vi "Measurement UI.vi"() -> ()   [LabVIEW 2021, in "Quiescent Current_Channel Ganging_UI.lvlib"]
uses:
  Quiescent Current_Channel Ganging_UI.lvlib
panel:
  in  "MeasGraphs":enum32{"Q Current", "Hidden Controls"}(tab)
  out "QCurrentGraph(V/A)":T1(graph)
  in  "Source voltage pole-zero ratio":dbl=2.0
  in  "Source voltage compensation frequency":dbl=3530.0
  in  "Source voltage gain bandwidth":dbl=2000.0
  out "Q current minimum":dbl
  out "Q current maximum":dbl
  out "Ganged q currents":dbl[](array[numeric]) caption="Q currents"
  out "Ganged source voltages":dbl[](array[numeric]) caption="Source voltages"
  in  "Source slave resource names":string[](array[string])
  in  "Source master resource name":string
  out "MeasTable":string[][](table)
  in  "MeasConfigurations":enum32{"Measurement Config", "Source Config"}(tab)=enum."Source Config"
  in  "Source delay":dbl=0.005 caption="SOURCE DELAY" format="%.3ps"
  in  "DUT setup time":dbl=1.0 caption="DUT SETUP TIME" format="%.3ps"
  in  "Aperture time":dbl=0.005 caption="APERTURE TIME" format="%.3ps"
  in  "PPSSlaveResourceNames":refnum<k15>[](array[refnum]) caption="SLAVE RESOURCE NAMES"
  in  "PPSMasterResourceName":refnum<k15> caption="MASTER RESOURCE NAME"
  in  "Source stop voltage":dbl=14.0 caption="VOLTAGE STOP LEVEL" format="%#_6pV"
  in  "Source transient response":i32(ring)=1038 caption="TRANSIENT RESPONSE" items=["Slow"=1041, "Normal"=1038, "Fast"=1039, "Custom"=1042]
  in  "Source sense":i32(ring)=1009 caption="SENSE" items=["Local"=1008, "Remote"=1009]
  in  "Source voltage level range":dbl=20.0 caption="VOLTAGE LEVEL RANGE" format="%#_6pV"
  in  "Source start voltage":dbl=6.0 caption="VOLTAGE START LEVEL" format="%#_6pV"
  in  "Source current limit high":dbl=25.0 caption="CURRENT LIMIT/LIMIT HIGH" format="%#_6pA"
  in  "Source current limit range":dbl=25.0 caption="CURRENT LIMIT RANGE" format="%#_6pA"
  in  "Source limit symmetry":enum32{"Symmetric", "Asymmetric"}(ring)=enum."Asymmetric" caption="LIMIT SYMMETRY"
  in  "Source current limit low":dbl=-0.6 caption="CURRENT LIMIT LOW" format="%#_6pA"
  in  "Source system configuration":enum32{"Series", "Parallel"}(ring)=enum."Parallel" caption="SYSTEM CONFIG"
  in  "Source compliance":string="Compliance"
  in  "Source sourceadapt":string="SourceAdapt"
  in  "Source Custom Transient Response":bool
  in  "Source voltage sweep points":i32=10 caption="SWEEP POINTS"
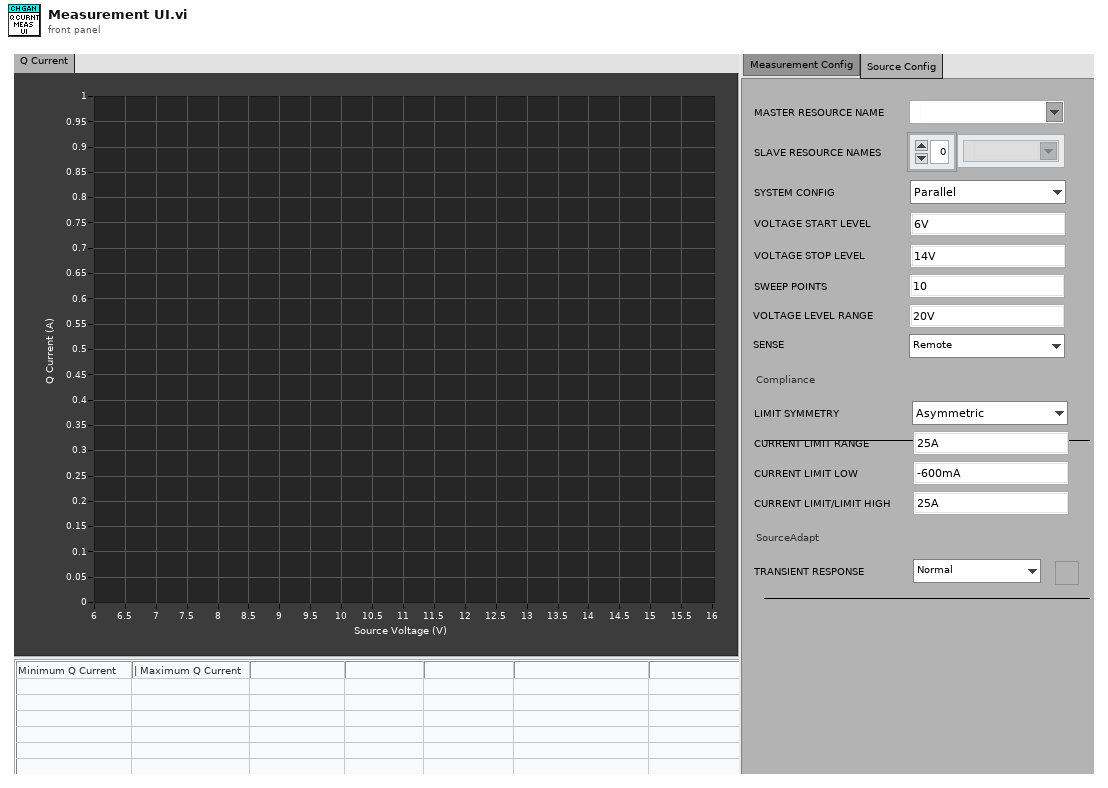
[diagram p1: front panel]
types:
  T1 = cluster{"Source voltages":dbl[], "Load voltages":dbl[]}
  T2 = typedef "SourceAdapt Parameters.ctl" = cluster{"Voltage gain bandwidth":dbl, "Voltage compensation frequency":dbl, "Voltage pole-zero ratio":dbl, "Current gain bandwidth":dbl, "Current compensation frequency":dbl, "Current pole-zero ratio":dbl}
  T3 = cluster{"Ganged source voltages":dbl[], "Ganged q currents":dbl[]}
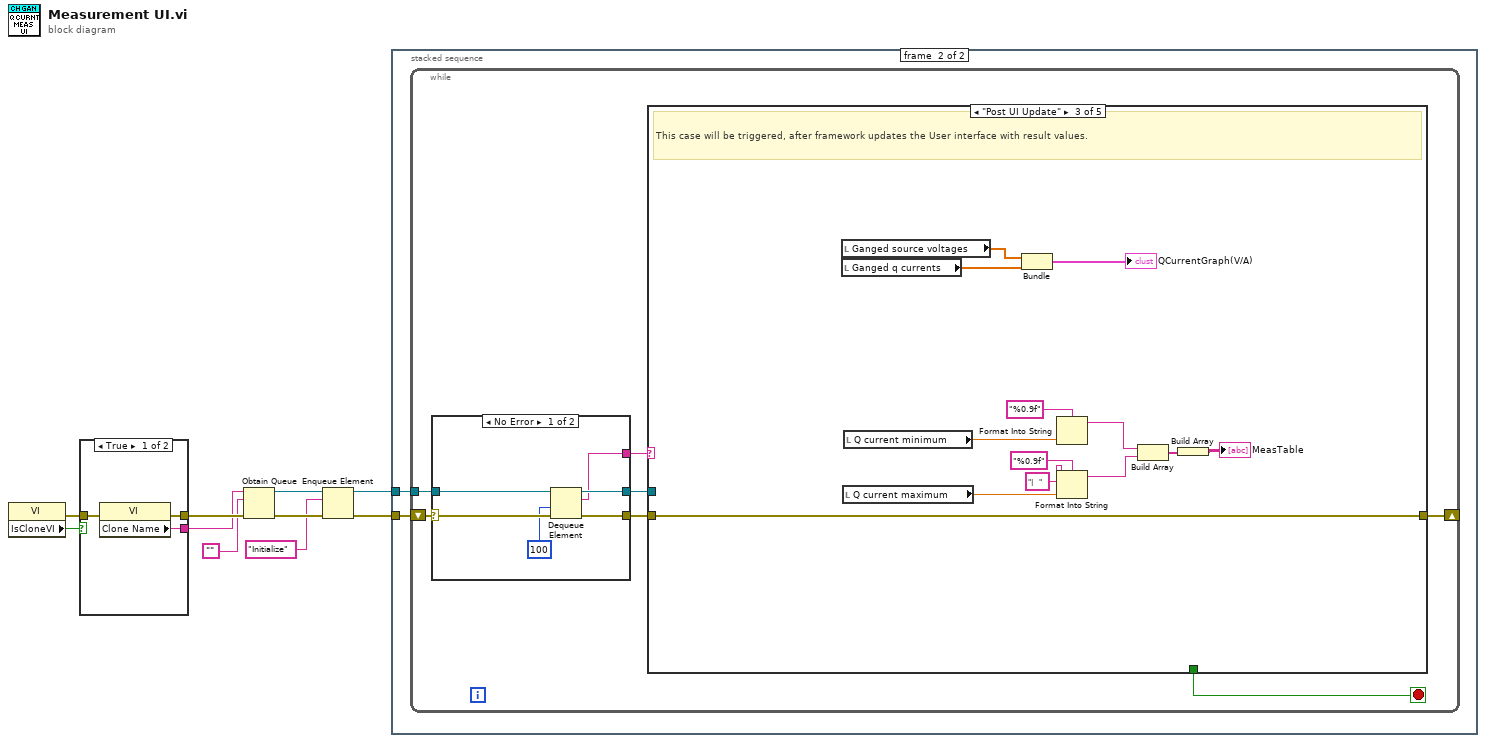
[diagram p0: block diagram]
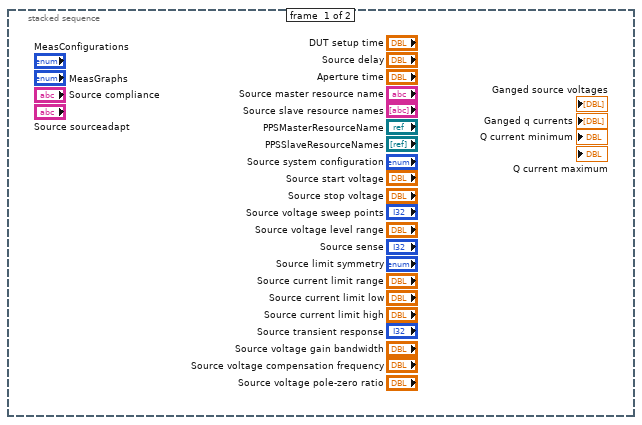
[diagram p2: hidden frame]
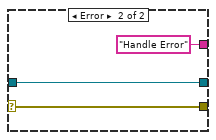
[diagram p3: hidden frame]
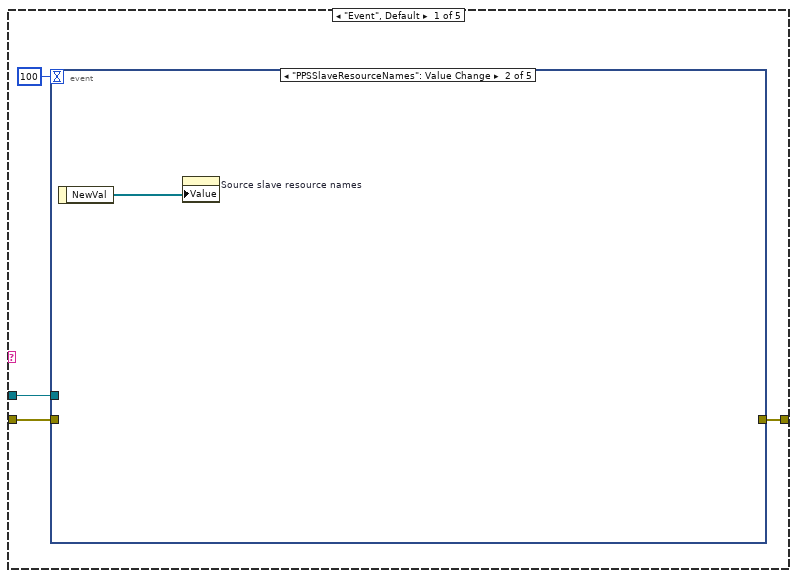
[diagram p4: hidden frame]
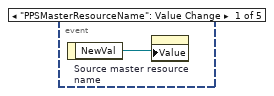
[diagram p5: hidden frame]
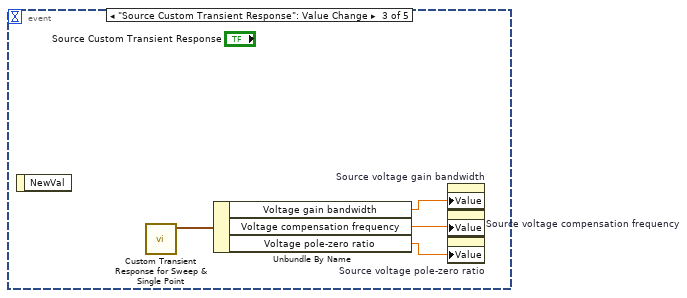
[diagram p6: hidden frame]
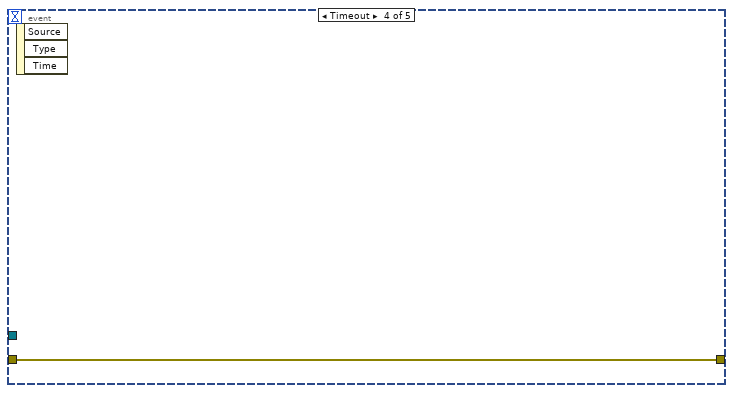
[diagram p7: hidden frame]
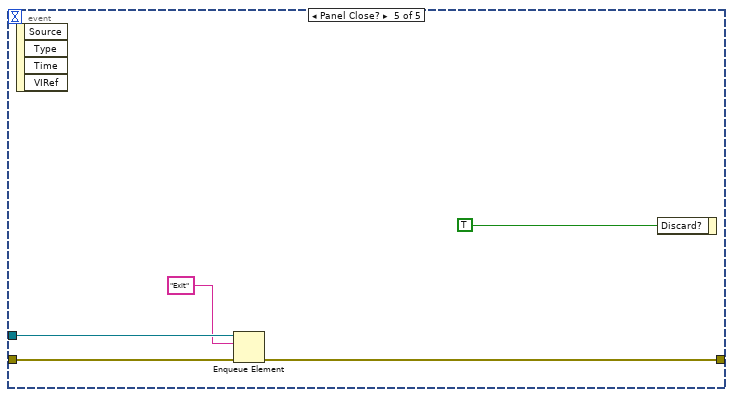
[diagram p8: hidden frame]
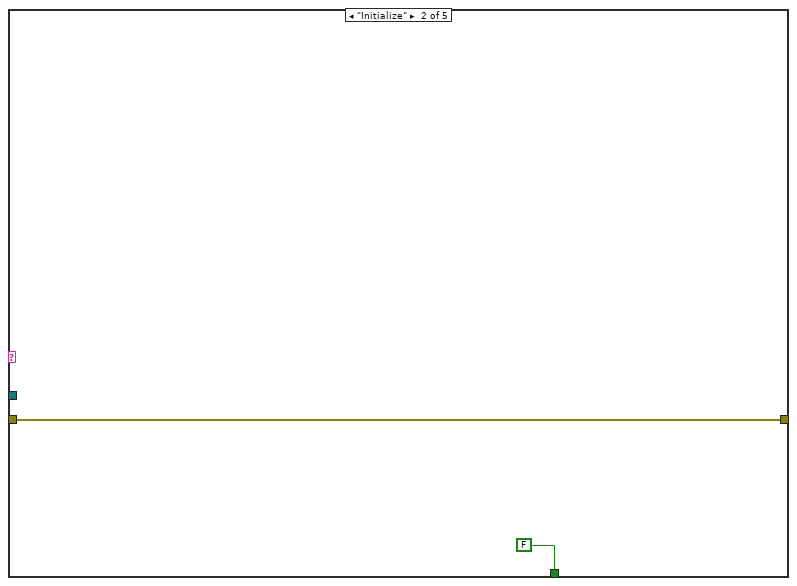
[diagram p9: hidden frame]
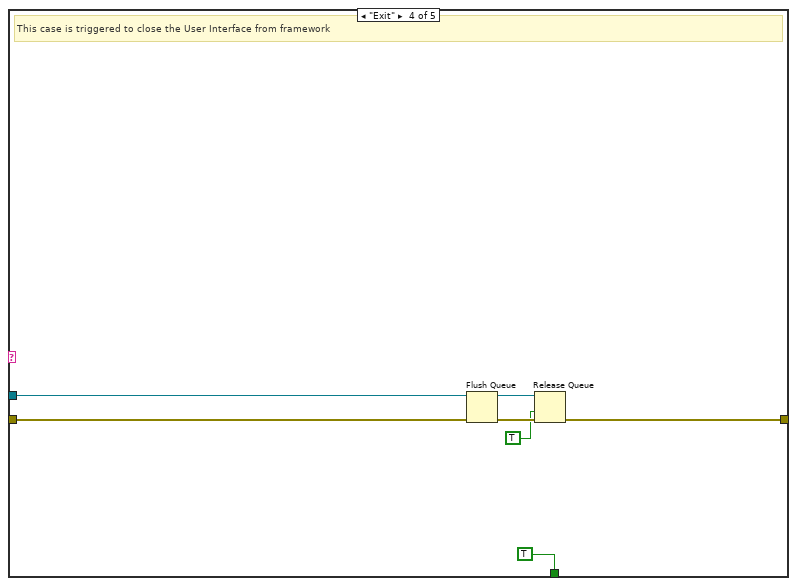
[diagram p10: hidden frame]
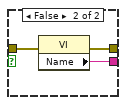
[diagram p12: hidden frame]
diagram:
  n1 = property class="VI"() -> (error out=w1:errorcluster, "IsCloneVI"=w2:bool)  [unwired: 2 in, 1 out]
  n2 = case shown="True" w2 {
    tunnel: [w13 w16] -> w10
    tunnel: [w12 w15] -> w9
    tunnel: w1 -> [w11 w14]
    frame True {
      n3 = property class="VI"(error in=w11) -> (error out=w13:errorcluster, "Clone Name"=w12:string)  [unwired: 1 in, 1 out]
    }
    frame False {
      n4 = property class="VI"(error in=w14) -> (error out=w16:errorcluster, "Name"=w15:string)  [unwired: 1 in, 1 out]
    }
  }
  n5 = Obtain Queue(name (unnamed)=w9, element data type="", error in (no error)=w10) -> (queue out=w6:refnum<queue>, error out=w8:errorcluster)  [unwired: 2 in, 1 out]
  n6 = Enqueue Element(queue=w6, element="Initialize", error in (no error)=w8) -> (queue out=w5:refnum<queue>, error out=w7:errorcluster)  [unwired: 1 in, 1 out]
  n7 = stacked-sequence {
    tunnel: w7 -> [_ w18]
    tunnel: w5 -> [_ w17]
    frame #0 {
    }
    frame #1 {
      n8 = while {
        shift-right: [w20] -> _
        shift-left: w18 -> [w25]
        tunnel: w17 -> [w23]
        stop <- w19 stop-if-true
        n9 = case shown="No Error" w25 {
          selector: w25 -> [w31 w34]
          tunnel: [w30 w34] -> w24
          tunnel: w23 -> [w29 w33]
          tunnel: [w28 w33] -> w22
          tunnel: [w27 "Handle Error"] -> w21
          frame No Error {
            n10 = Dequeue Element(queue=w29, timeout in ms (-1)=100, error in (no error)=w31) -> (queue out=w28:refnum<queue>, element=w27:string, error out=w30:errorcluster)  [unwired: 1 out]
          }
          frame Error {
          }
        }
        n11 = case shown="\"Post UI Update\"" w21 {
          tunnel: w24 -> [w37 w52 w65 w72 w73]
          tunnel: w22 -> [w35 _ _ w70 _]
          tunnel: [w38 w52 w65 w67 w73] -> w20
          tunnel: [_ FALSE _ TRUE _] -> w19
          frame "Event", Default {
            n12 = event shown="[1] \"PPSSlaveResourceNames\": Value Change" {
              selector: _ -> [_ _ _ _ _]
              dyn-events: _ -> [_ _ _ _ _]
              timeout: 100 -> [_ _ _ _ _]
              tunnel: [_ _ _ w45 w48] -> w38
              tunnel: w37 -> [_ _ _ w45 w49]
              tunnel: w35 -> [_ _ _ _ w47]
              event "PPSMasterResourceName": Value Change {
                n13 = event-data() -> ("NewVal"=w39:refnum<k15>)  [unwired: 1 in]
                n14 = property on="Source master resource name" class="Str"("Value"=w39) -> ()  [unwired: 2 in, 2 out]
              }
              event "PPSSlaveResourceNames": Value Change {
                n15 = event-data() -> ("NewVal"=w40:refnum<k15>[])  [unwired: 1 in]
                n16 = property on="Source slave resource names" class="Arr (strict)"("Value"=w40) -> ()  [unwired: 2 in, 2 out]
              }
              event "Source Custom Transient Response": Value Change {
                n17 = event-data() -> ()  [unwired: 1 in, 1 out]
                n18 = call "Custom Transient Response for Sweep & Single Point.vi"() -> ("SourceAdapt Parameters"=w44:T2)  [unwired: 11 in]
                n19 = Unbundle By Name(w44) -> ("Voltage gain bandwidth"=w43:dbl, "Voltage compensation frequency"=w42:dbl, "Voltage pole-zero ratio"=w41:dbl)
                n20 = property on="Source voltage gain bandwidth" class="DigNum (strict)"("Value"=w43) -> ()  [unwired: 2 in, 2 out]
                n21 = property on="Source voltage compensation frequency" class="DigNum (strict)"("Value"=w42) -> ()  [unwired: 2 in, 2 out]
                n22 = property on="Source voltage pole-zero ratio" class="DigNum (strict)"("Value"=w41) -> ()  [unwired: 2 in, 2 out]
              }
              event Timeout {
                n23 = event-data() -> ()  [unwired: 1 in, 3 out]
              }
              event Panel Close? {
                n24 = event-data() -> ()  [unwired: 1 in, 4 out]
                n25 = Enqueue Element(queue=w47, element="Exit", error in (no error)=w49) -> (error out=w48:errorcluster)  [unwired: 1 in, 2 out]
                n26 = event-data("Discard?"=TRUE) -> ()  [unwired: 1 in, 1 out]
              }
            }
          }
          frame "Initialize" {
          }
          frame "Post UI Update" {
            # "This case will be triggered, after framework updates the User interface with result values."
            n27 = local read "Ganged source voltages"() -> (w61:dbl[])
            n28 = local read "Ganged q currents"() -> (w60:dbl[])
            n29 = local read "Q current maximum"() -> (w58:dbl)
            n30 = local read "Q current minimum"() -> (w59:dbl)
            n31 = Bundle("Ganged source voltages"=w61, "Ganged q currents"=w60) -> (→"QCurrentGraph(V/A)":T3)  [unwired: 1 in]
            n32 = Format Into String(format string="%0.9f" ("initial string"), w59) -> (resulting string=w55:string)  [unwired: 2 in, 1 out]
            n33 = Format Into String(format string="%0.9f" ("initial string"), initial string="|   ", w58) -> (resulting string=w56:string)  [unwired: 1 in, 1 out]
            n34 = Build Array(w55, w56) -> (w57:string[])
            n35 = Build Array(w57) -> (→"MeasTable":string[][])
          }
          frame "Exit" {
            # "This case is triggered to close the User Interface from framework"
            n36 = Flush Queue(queue=w70, error in (no error)=w72) -> (queue out=w69:refnum<queue>, error out=w68:errorcluster)  [unwired: 1 out]
            n37 = Release Queue(queue=w69, force destroy? (F)=TRUE, error in (no error)=w68) -> (error out=w67:errorcluster)  [unwired: 2 out]
          }
          frame "Handle Error" {
          }
        }
      }
    }
  }
